vi "kinetic simulation matrix-2.vi"() -> ()   [LabVIEW 2012]
uses:
  <vilib>/Utility/file.llb/Write To Spreadsheet File (DBL).vi
panel:
  out "Simulated-Efficencys":dbl[][](array[numeric])=[[90.8309887459807, 91.11233922829581, 91.11233922829581, 91.11233922829581, 91.11233922829581], [79.0, 86.0, 93.0, 96.0, 97.0], [88.0, 90.0, 91.0, 92.0, 90.0], [91.0, 90.0, 90.0, 91.0, 90.0]]
  in  "State to Observe":i32=4
  in  "incubation time":dbl[](array[numeric])=[30.0, 100.0, 300.0, 1000.0, 3000.0] caption="Incubation time"
  in  "concentration (uM)":dbl[](array[numeric])=[0.2, 0.5, 1.0, 10.0]
  in  "Experamental-Efficencys":dbl[][](array[numeric])=[[70.0, 85.0, 91.0, 95.0, 99.0], [79.0, 86.0, 93.0, 96.0, 97.0], [88.0, 90.0, 91.0, 92.0, 90.0], [91.0, 90.0, 90.0, 91.0, 90.0]]
  out "Efficency Summery":dbl[][](graph)=[[70.0, 85.0, 91.0, 95.0, 99.0], [79.0, 86.0, 93.0, 96.0, 97.0], [88.0, 90.0, 91.0, 92.0, 90.0], [91.0, 90.0, 90.0, 91.0, 90.0], [64.6875, 86.875, 99.0625, 99.6875, 99.6875], [78.16901408450704, 97.53521126760563, 98.76760563380282, 98.76760563380282, 98.76760563380282], [88.84514435695539, 98.16272965879264, 98.16272965879264, 98.16272965879264, 98.16272965879264], [90.8309887459807, 91.11233922829581, 91.11233922829581, 91.11233922829581, 91.11233922829581]]
  in  "k2":dbl=0.14 format="%#_6f"
  in  "AF/F":bool=TRUE
  in  "Matrix-Antifuel":dbl[][](array[numeric])=[[0.0, 0.0, 0.0, 0.0, 0.0, 0.0, 0.0, 0.0, 0.0, 0.0], [0.0, 0.0, 0.0, 0.0, 0.0, 0.0, 0.0, 0.0, 0.0, 0.0], [0.0, 0.0, 0.0, 0.0, 0.0, 0.0, 0.0, 0.0, 0.0, 0.0], [0.0, 0.0, 0.0, 0.0, 0.0, 0.0, 0.0, 0.0, 0.0, 0.0], [0.75, 0.0, 0.0, 0.0, 0.0, 0.0, 0.0, 0.0, 0.0, 0.0], [0.0, 0.0, 0.0, 0.0, 0.0, 0.0, 0.0, 0.0, 0.0, 0.0]]
  out "Concen (um)":dbl=10.0
  in  "kF (um)":dbl=0.075 format="%#_6f"
  out "Efficency (end)":dbl[](array[numeric])=[0.0, 0.0, 0.0, 0.17783582839344922, 0.8222646438259821]
  out "kF'X":dbl=0.026250000000000002
  in  "X":dbl=0.035
  out "kF'":dbl=0.75
  out "nnew 2":i32=1
  out "inew 2":i32=1
  out "index_top 2":i32=2
  out "Final_A_index 2":i32[](array[numeric])=[0, 1, 2, 5, 2, 0, 0, 0, 0, 0]
  out "Final_D_index 2":i32[](array[numeric])=[0, 2, 1, 1, 4, 0, 0, 0, 0, 0]
  out "rate 2":dbl[](array[numeric])=[0.0, 0.0, 0.0, 0.0, 4000000000.000001, 0.0, 0.0, 0.0, 0.0, 0.0]
  in  "Matrix-Fuel":dbl[][](array[numeric])=[[0.0, 0.0, 0.0, 0.0, 0.0, 0.0, 0.0, 0.0, 0.0, 0.0], [0.75, 0.0, 0.0, 0.0, 0.0, 0.0, 0.0, 0.0, 0.0, 0.0], [0.026250000000000002, 0.0, 0.0, 0.0, 0.0, 0.0, 0.0, 0.0, 0.0, 0.0], [0.0, 0.026250000000000002, 0.75, 0.0, 0.0, 0.0, 0.0, 0.0, 0.0, 0.0], [0.0, 0.14, 0.14, 0.0, 0.0, 0.0, 0.0, 0.0, 0.0, 0.0], [0.0, 0.0, 0.0, 0.0, 0.0, 0.0, 0.0, 0.0, 0.0, 0.0]]
  in  "save?":bool
  out "nnew":i32=1
  out "inew":i32=1
  out "index_top":i32=2
  out "photime":dbl=9999.0
  out "srate":dbl
  out "time 2":dbl=0.30115000000000003
  out "Final_A_index":i32[](array[numeric])=[0, 1, 2, 5, 2, 0, 0, 0, 0, 0]
  out "Final_D_index":i32[](array[numeric])=[0, 2, 1, 1, 4, 0, 0, 0, 0, 0]
  out "rate":dbl[](array[numeric])=[0.0, 0.0, 0.0, 0.0, 333333000.0, 0.0, 0.0, 0.0, 0.0, 0.0]
  out "X-axes":dbl[](array[numeric])
  in  "time max":dbl=3000.0
  out "Kinetics":dbl[][](graph)
  in  "time per bin":dbl=0.1
  in  "NEXT":bool
  in  "number of state obs":i32=5
  out "Current pos":i32=5
  in  "start pos":i32
  out "probabilty distribution":dbl[](graph)=[12822.454694565015, 57004.60141146341, 400.51524158787134, 5298639.656530077, 24493132.772122297, 0.0, 0.0, 0.0, 0.0, 0.0, 0.0, 0.0, 0.0]
  out "time":dbl=3000.0 format="%.3e"
  in  "stop inside":bool
  # "B"
  # "B"
  # "C'"
  # "D"
  # "C'"
  # "D"
  # "A"
  # "B'"
  # "A"
  # "B'"
  # "A"
  # "A"
  # "B"
  # "B"
  # "B'"
  # "B'"
  # "C'"
  # "FUEL"
  # "kF'"
  # "C'"
  # "D"
  # "D"
  # "ANTI-FUEL"
  # "kF'x"
  # "kF'x"
  # "kF'"
  # "k2"
  # "k2"
  # "200 nM"
  # "500 nM"
  # "1 uM"
  # "10 uM"
  # "30s"
  # "300s"
  # "3000s"
  # "100s"
  # "1000s"
  # "k1 B->D"
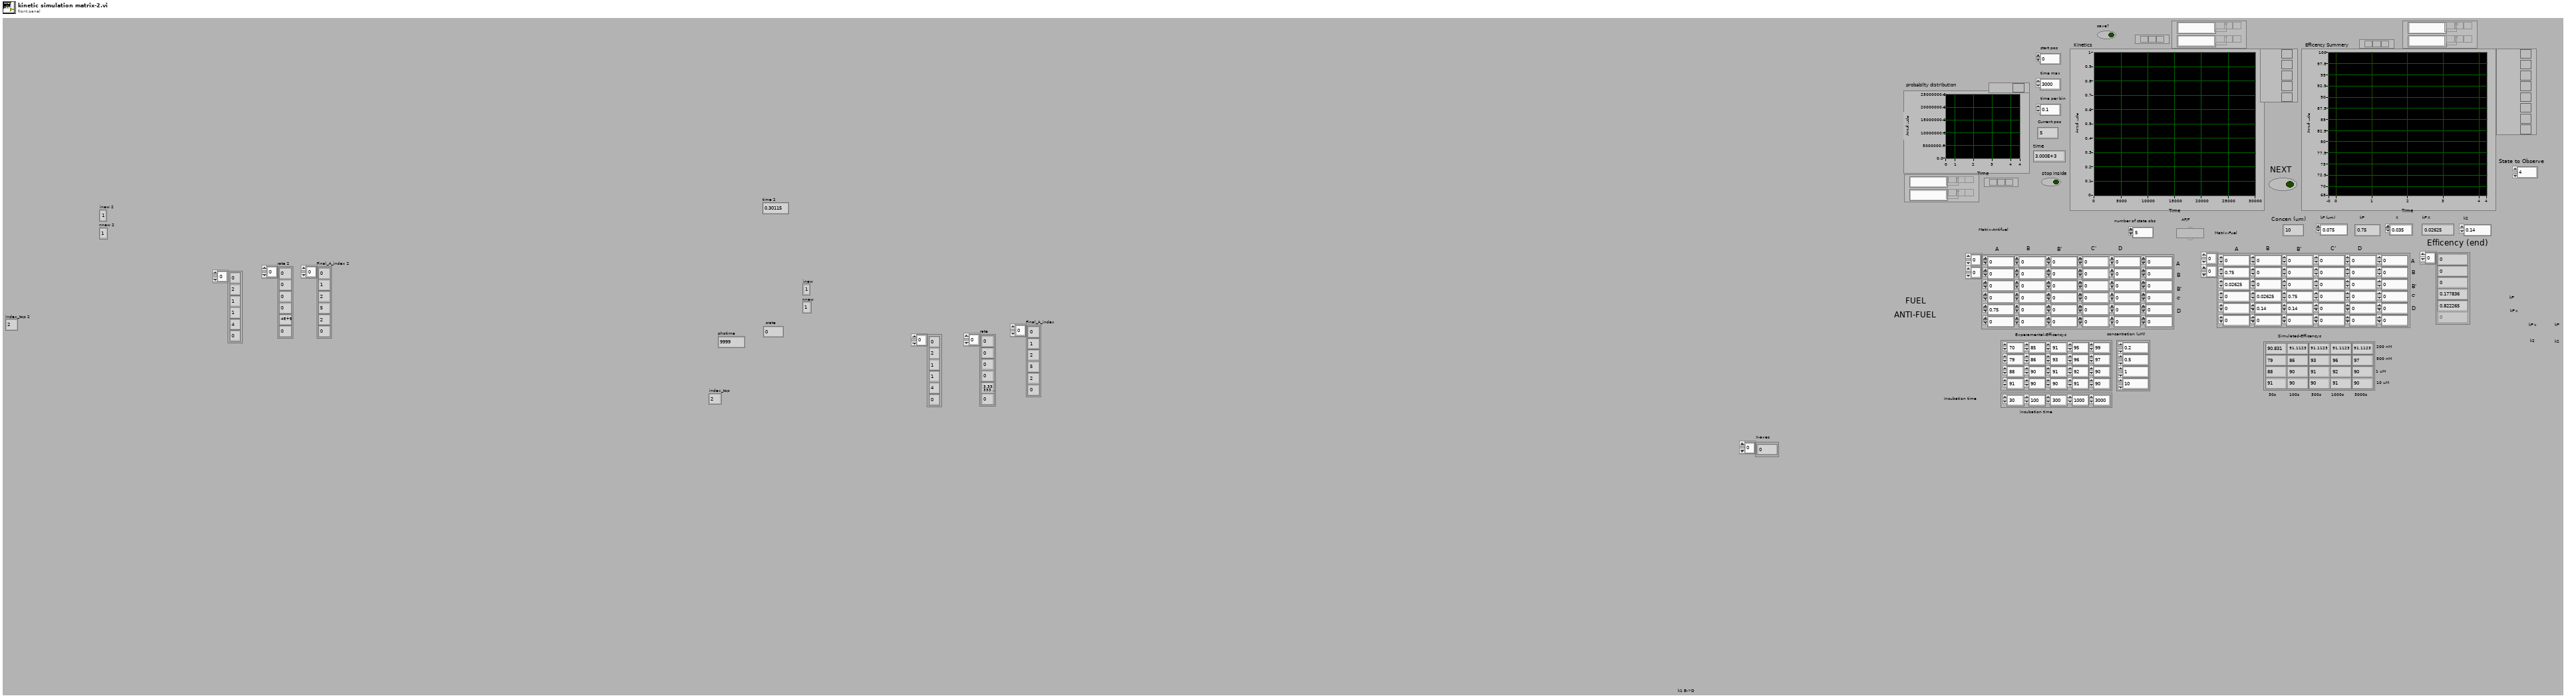
[diagram p1: front panel]
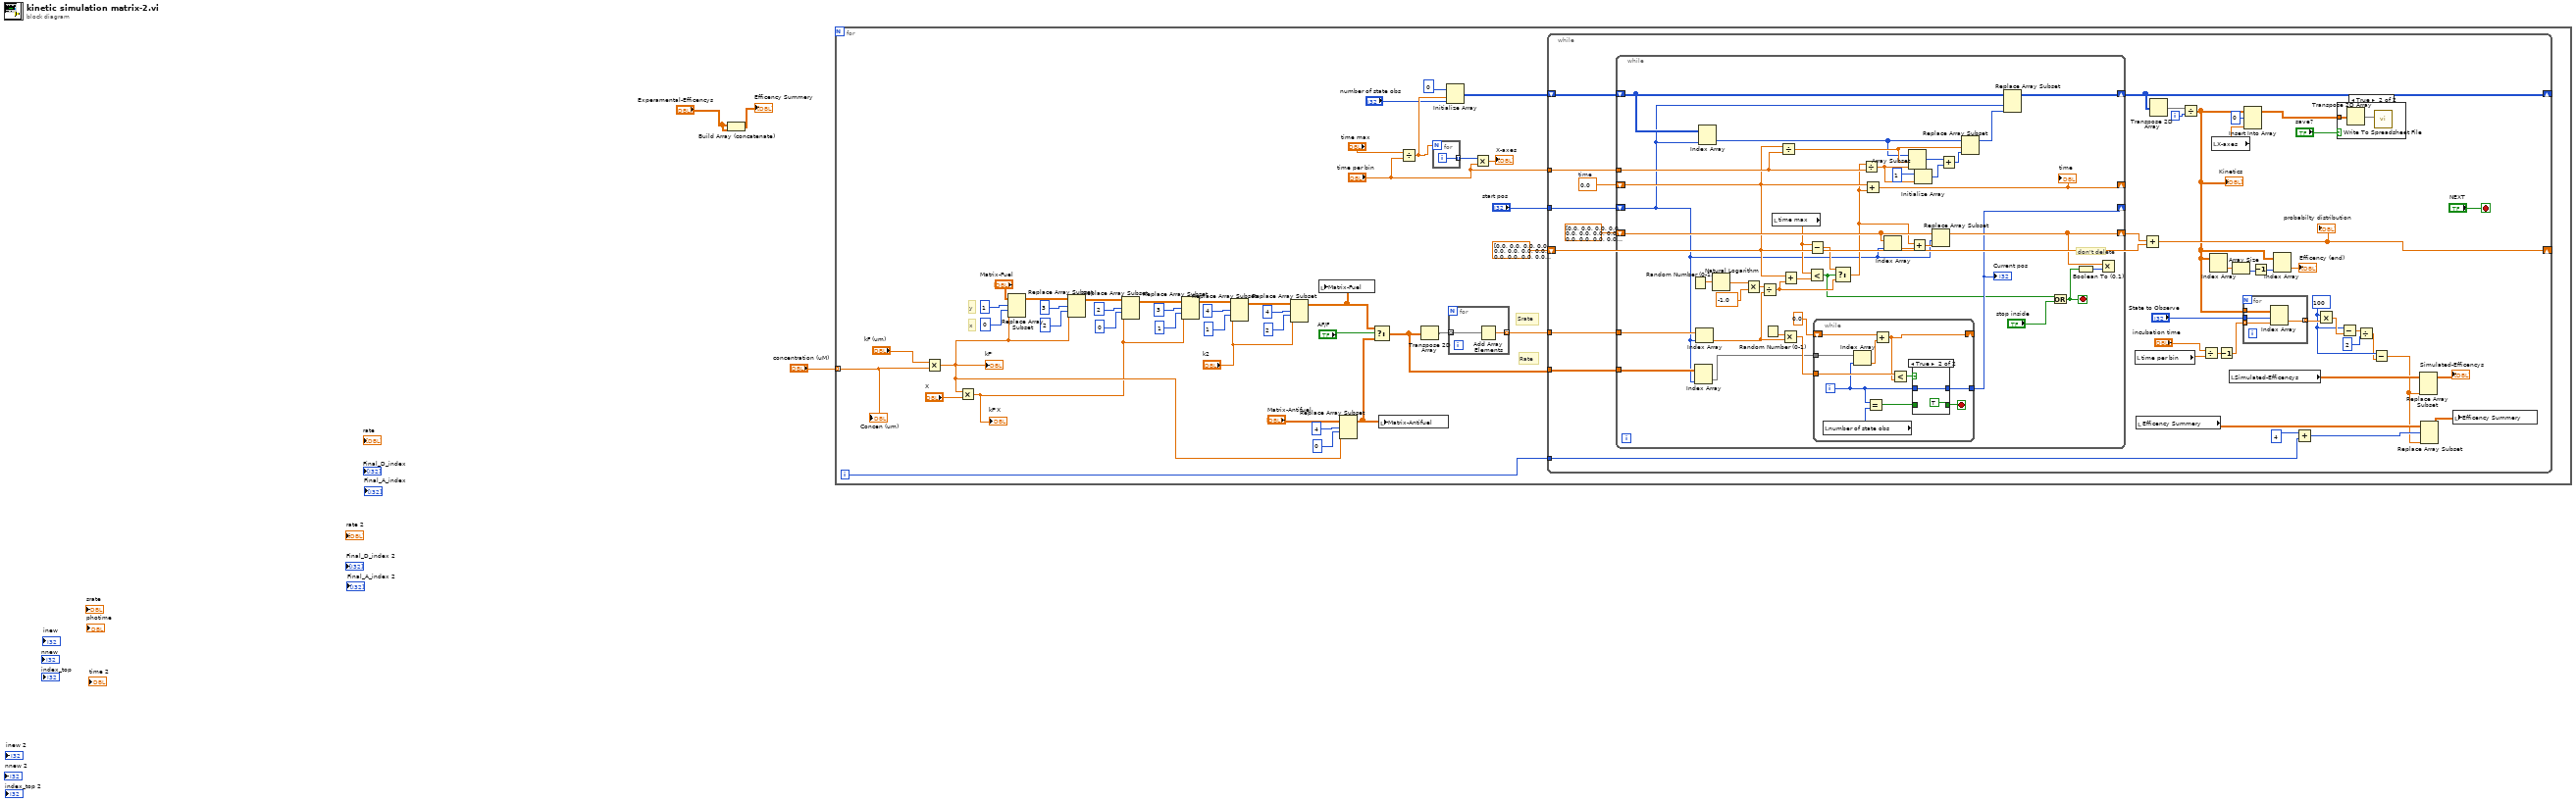
[diagram p0: block diagram]
diagram:
  n1 = Build Array (concatenate)("Experamental-Efficencys", "Experamental-Efficencys") -> (→"Efficency Summery":dbl[][])
  n2 = for {
    tunnel: "concentration (uM)" -> [w5] mode=indexing
    i -> [w4]
    # "y"
    # "x"
    # "Rate"
    # "Srate"
    n3 = Multiply(x="kF (um)", y=w5) -> (x*y=w7:dbl)
    "kF'" <- w7
    n4 = Multiply(x=w7, y="X") -> (x*y=w6:dbl)
    "kF'X" <- w6
    n5 = Replace Array Subset(array="Matrix-Fuel", new element=w7, index (row)=1, index (col)=0 ("disabled index (col)")) -> (w27:dbl[][])
    n6 = Replace Array Subset(array=w27, new element=w7, index (row)=3, index (col)=2 ("disabled index (col)")) -> (w21:dbl[][])
    n7 = Replace Array Subset(array=w21, new element=w6, index (row)=2, index (col)=0 ("disabled index (col)")) -> (w22:dbl[][])
    n8 = Replace Array Subset(array=w22, new element=w6, index (row)=3, index (col)=1 ("disabled index (col)")) -> (w15:dbl[][])
    n9 = Replace Array Subset(array=w15, new element="k2", index (row)=4, index (col)=1 ("disabled index (col)")) -> (w16:dbl[][])
    n10 = Replace Array Subset(array=w16, new element="k2", index (row)=4, index (col)=2 ("disabled index (col)")) -> (w12:dbl[][])
    n11 = local write "Matrix-Fuel"(w12) -> ()
    n12 = Replace Array Subset(array="Matrix-Antifuel", new element=w7, index (row)=4, index (col)=0 ("disabled index (col)")) -> (w8:dbl[][])
    n13 = Select(t=w12, s="AF/F", f=w8) -> (s? t:f=w35:dbl[][])
    n14 = local write "Matrix-Antifuel"(w8) -> ()
    n15 = Divide(x="time max", y="time per bin") -> (x/y=w44:dbl)
    n16 = Transpose 2D Array(2D array=w35) -> (transposed array=w39:dbl[][])
    n17 = for {
      N: w44 -> [_]
      tunnel: [w50] -> w41 mode=indexing
      i -> [w50]
    }
    n18 = Initialize Array(0 ("dimension size"), w44, "number of state obs") -> (w40:i32[][])
    n19 = for {
      tunnel: w39 -> [w48] mode=indexing
      tunnel: [w49] -> w38 mode=indexing
      n20 = Add Array Elements(numeric array=w48) -> (sum=w49:dbl)
    }
    n21 = Multiply(x=w41, y="time per bin") -> (x*y=→"X-axes":dbl[])
    n22 = while {
      shift-right: [w77] -> _
      shift-left: dbl[] [0.0, 0.0, 0.0, 0.0, 0.0, 0.0, 0.0, 0.0, 0.0, 0.0, 0.0, 0.0, 0.0] ("Output Array") -> [w91]
      tunnel: "time per bin" -> [w88]
      shift-right: [w85] -> _
      shift-left: w40 -> [w89]
      tunnel: w38 -> [w79]
      tunnel: w35 -> [w78]
      tunnel: "start pos" -> [w76]
      tunnel: w4 -> [w59]
      i -> [w75]
      stop <- "NEXT" stop-if-true
      w53 = 100 ("index (row)")
      w87 = 0.0  # time
      n23 = while {
        shift-left: dbl[] [0.0, 0.0, 0.0, 0.0, 0.0, 0.0, 0.0, 0.0, 0.0, 0.0, 0.0, 0.0, 0.0] ("Output Array") -> [w132]
        shift-right: [w111] -> w84
        shift-left: w87 -> [w114]
        shift-right: [w109] -> _
        shift-left: w76 -> [w104]
        shift-right: [w100] -> _
        tunnel: w88 -> [w125]
        shift-right: [w112] -> w85
        shift-left: w89 -> [w118]
        tunnel: w79 -> [w106]
        tunnel: w78 -> [w105]
        stop <- w129 stop-if-true
        # "don't delete"
        n24 = Random Number (0-1)() -> (number: 0 to 1=w137:dbl)
        n25 = Index Array(array=w105, index (col)=w104) -> (element=w101:dbl[])  [unwired: 1 in]
        n26 = Index Array(array=w106, index=w104) -> (element=w107:dbl)
        n27 = Index Array(array=w118, index (col)=w104) -> (element=w119:i32[])  [unwired: 1 in]
        n28 = Natural Logarithm(1:w137) -> (0:w136:dbl)
        n29 = Multiply(x=w136, y=-1.0) -> (x*y=w134:dbl)
        n30 = Divide(x=w134, y=w107) -> (x/y=w108:dbl)
        n31 = Random Number (0-1)() -> (number: 0 to 1=w133:dbl)
        n32 = local read "time max"() -> (w115:dbl)
        n33 = Divide(x=w114, y=w125) -> (x/y=w121:dbl)
        n34 = Multiply(x=w133, y=w107) -> (x*y=w102:dbl)
        n35 = Add(x=w114, y=w108) -> (x+y=w116:dbl)
        n36 = Less?(x=w115, y=w116) -> (x < y?=w99:bool)
        n37 = Subtract(x=w115, y=w114) -> (x-y=w113:dbl)
        n38 = while {
          shift-right: [w144] -> _
          shift-left: 0.0 -> [w147]
          tunnel: w102 -> [w145]
          tunnel: w101 -> [w141]
          tunnel: [w138] -> w100
          i -> [w140]
          stop <- w142 stop-if-true
          n39 = local read "number of state obs"() -> (w139:i32)
          n40 = Index Array(array=w141, index=w140) -> (element=w148:dbl)
          n41 = Equal?(x=w140, y=w139) -> (x = y?=w143:bool)
          n42 = Add(x=w147, y=w148) -> (x+y=w144:dbl)
          n43 = Less?(x=w145, y=w144) -> (x < y?=w146:bool)
          n44 = case shown="True" w146 {
            tunnel: w140 -> [w149 w151]
            tunnel: w143 -> [w150 _]
            tunnel: [w150 TRUE] -> w142
            tunnel: [w149 w151] -> w138
            frame False {
            }
            frame True {
            }
          }
        }
        "Current pos" <- w100
        n45 = Select(t=w113, s=w99, f=w108) -> (s? t:f=w110:dbl)
        n46 = Divide(x=w110, y=w125) -> (x/y=w120:dbl)
        n47 = Add(x=w114, y=w110) -> (x+y=w109:dbl)
        "time" <- w109
        n48 = Index Array(array=w132, index=w104) -> (element=w130:dbl)
        n49 = Array Subset(array=w119, index=w121, length=w120) -> (w124:i32[])
        n50 = Add(x=w110, y=w130) -> (x+y=w131:dbl)
        n51 = Initialize Array(1 ("dimension size"), w120) -> (w123:i32[])
        n52 = Replace Array Subset(array=w132, new element=w131, index=w104) -> (w111:dbl[])
        n53 = Add(x=w124, y=w123) -> (x+y=w122:i32[])
        n54 = Replace Array Subset(array=w119, new element=w122, index=w121) -> (w117:i32[])
        n55 = Replace Array Subset(array=w118, new element=w117, index (col)=w104) -> (w112:i32[][])  [unwired: 1 in]
        n56 = Or(x=w99, y="stop inside") -> (x .or. y?=w129:bool)
        n57 = Boolean To (0,1)(Boolean=w129) -> (0, 1=w128:i16)
        n58 = Multiply(x=w111, y=w128) -> ()  [unwired: 1 out]
      }
      n59 = local read "time per bin"() -> (w67:dbl)
      n60 = local read "Efficency Summery"() -> (w60:dbl[][])
      n61 = Add(x=w84, y=w91) -> (x+y=w77:dbl[])
      "probabilty distribution" <- w77
      n62 = Transpose 2D Array(2D array=w85) -> (transposed array=w86:i32[][])
      n63 = Divide(x=w86, y=w75) -> (x/y=w68:dbl[][])
      "Kinetics" <- w68
      n64 = Divide(x="incubation time", y=w67) -> (x/y=w66:dbl[])
      n65 = Index Array(array=w68) -> (element=w71:dbl[])  [unwired: 2 in]
      n66 = local read "X-axes"() -> (w80:dbl[])
      n67 = Decrement(x=w66) -> (x-1=w64:dbl[])
      n68 = local read "Simulated-Efficencys"() -> (w74:dbl[][])
      n69 = Array Size(array=w71) -> (size(s)=w69:i32)
      n70 = for {
        tunnel: w64 -> [w96] mode=indexing
        tunnel: [w95] -> w63 mode=indexing
        tunnel: "State to Observe" -> [w94]
        tunnel: w68 -> [w93]
        n71 = Index Array(array=w93, index (row)=w94, index (col)=w96) -> (element=w95:dbl)
      }
      n72 = Insert Into Array(array=w68, index (row)=0, new element=w80) -> (w82:dbl[][])  [unwired: 1 in]
      n73 = Decrement(x=w69) -> (x-1=w70:i32)
      n74 = Index Array(array=w68, index (col)=w70) -> (element=→"Efficency (end)":dbl[])  [unwired: 1 in]
      n75 = Add(x=4 ("index (row)"), y=w59) -> (x+y=w57:i32)
      n76 = Multiply(x=w53, y=w63) -> (x*y=w56:dbl[])
      n77 = case shown="True" "save?" {
        tunnel: w82 -> [_ w98]
        frame False {
        }
        frame True {
          n78 = Transpose 2D Array(2D array=w98) -> (transposed array=w97:dbl[][])
          n79 = call-poly <vilib>:"Write To Spreadsheet File.vi"("2D data"=w97) -> ()  [unwired: 7 in, 1 out]
        }
      }
      n80 = Subtract(x=w53, y=w56) -> (x-y=w55:dbl[])
      n81 = Divide(x=w55, y=2 ("index (row)")) -> (x/y=w52:dbl[])
      n82 = Subtract(x=w53, y=w52) -> (x-y=w51:dbl[])
      n83 = Replace Array Subset(array=w74, new element=w51) -> (→"Simulated-Efficencys":dbl[][])  [unwired: 2 in]
      n84 = Replace Array Subset(array=w60, new element=w51, index (row)=w57) -> (w61:dbl[][])  [unwired: 1 in]
      n85 = local write "Efficency Summery"(w61) -> ()
    }
    "Concen (um)" <- w5
  }
